vi "Memory Init.vi"(8 "Wave path":path) -> ()   [LabVIEW 2014]
uses:
  <vilib>/Utility/error.llb/Clear Errors.vi
  <vilib>/rvi/Emulation/niFpgaSctlEmulationGetInTimedLoop.vi
  <vilib>/Utility/file.llb/Read From Spreadsheet File (I64).vi
  <vilib>/rvi/Memory/Memory_Emulation/nirvimemoryEmulation.vi
  <vilib>/rvi/Memory/Memory_Emulation/nirvimemoryFastEmulation.vi
  <vilib>/rvi/DataTransferAndStorage/Container/Common/niFpgaContainerGetUniqueNameForEmu.vi
  <vilib>/rvi/Memory/Memory_Emulation/niFpgaMemoryEmulationCacheClearOnFirstRun.vi
  <vilib>/rvi/Memory/Memory_Emulation/nirvimemoryEmulationManagerCache_MakeExclusive.vi
  <vilib>/rvi/Memory/Memory_Emulation/niFpgaMemoryEmulationValidateCache.vi
  <vilib>/rvi/Memory/Memory_Emulation/nirvimemoryEmulationManagerCache_InsertValue.vi
  <vilib>/rvi/Memory/Memory_Emulation/nirvimemoryEmulationManagerCache_ReleaseExclusive.vi
  <vilib>/rvi/Memory/Memory_Emulation/nirvimemoryEmulationManagerCache_GetValue.vi
  <vilib>/rvi/Emulation/niFpgaEmulationIsFPGAContextNoSignature.vi
  <vilib>/rvi/Memory/Memory_Emulation/nirvimemoryEmulationManagerCache_SetValue.vi
  <vilib>/rvi/Emulation/niFpgaSctlEmulationResourceMgr.vi
  <vilib>/rvi/DataTransferAndStorage/Container/XNode/niFpgaContainer.xnode
panel:
  in  "File name":string
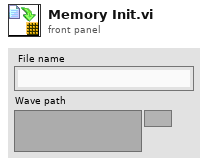
[diagram p1: front panel]
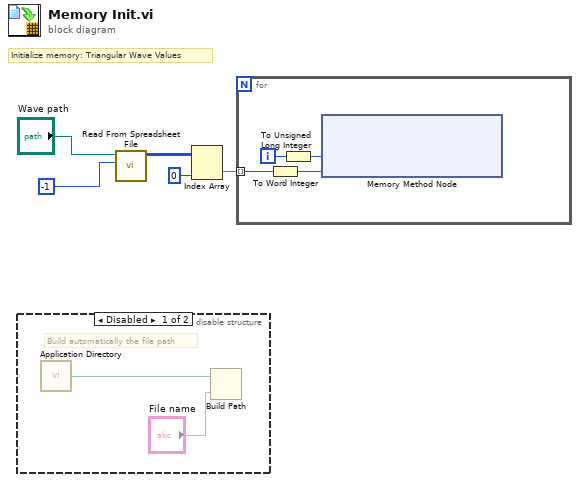
[diagram p0: block diagram]
diagram:
  # "Initialize memory: Triangular Wave Values"
  n1 = disable-structure shown="Disabled" {
    frame Disabled {
      # "Build automatically the file path"
      n2 = call <vilib>:"Application Directory.vi"() -> ("Application Directory"=w7:path)
      n3 = Build Path(base path=w7, name or relative path="File name") -> ()  [unwired: 1 out]
    }
    frame Enabled {
    }
  }
  n4 = call-poly <vilib>:"Read From Spreadsheet File.vi"("number of rows (all:-1)"=-1, "file path (dialog if empty)"="Wave path") -> ("all rows"=w4:i64[][])  [unwired: 5 in, 4 out]
  n5 = Index Array(array=w4, index (col)=0 ("disabled index (col)")) -> (element=w2:i64[])  [unwired: 1 in]
  n6 = for {
    tunnel: w2 -> [w11] mode=indexing
    i -> [w9]
    n7 = To Word Integer(number=w11) -> (16bit integer=w10:i16)
    n8 = To Unsigned Long Integer(number=w9) -> (unsigned 32bit integer=w8:u32)
    n9 = xnode ("Memory Method Node")("Address"=w8, "Data"=w10) -> ()  [unwired: 1 in, 1 out]
  }
